vi "DBtest.vi"() -> ()   [LabVIEW 2010]
uses:
  <vilib>/addons/database/Connection.llb/DB Tools Open Connec (Path).vi
  70user.lib/TheSigTab.vi
  <vilib>/addons/database/Connection.llb/Conn Get Properties.vi
  <vilib>/addons/database/NI_Database_API.lvlib
panel:
  out "provider":string
  in  "AllMeasures":cluster{"x0":dbl, "dx":dbl, "y":sgl[][]}[](array[cluster])=[{"x0"=0.0, "dx"=2.011173184357542, "y"=[7.555169582366943, 7.5977783203125, 7.770636558532715, 7.640630722045898, 7.5977783203125, 7.9028544425964355, 7.512796401977539, 7.555169582366943, 7.533955097198486, 7.345677375793457, 7.4496870040893555, 7.640630722045898, 7.491700649261475, 7.387104511260986, 7.576444149017334, 7.263514995574951, 7.512796401977539, 7.576444149017334, 7.263514995574951, 7.814460277557373, 7.662145614624023, 7.512796401977539, 7.3250508308410645, 7.79251766204834, 7.576444149017334, 8.105413436889648, 7.4706645011901855, 7.4496870040893555, 7.407908916473389, 7.705357551574707, 7.6191725730896, 7.555169582366943, 7.345677375793457, 7.662145614624023, 7.662145614624023, 7.4496870040893555, 7.407908916473389, 7.836464881896973, 7.4706645011901855, 7.283968448638916, 7.491700649261475, 7.640630722045898, 7.4496870040893555, 7.662145614624023, 7.705357551574707, 7.533955097198486, 7.283968448638916, 7.9028544425964355, 7.555169582366943, 7.8806633949279785, 7.683721542358398, 7.836464881896973, 7.727055072784424, 7.512796401977539, 7.576444149017334, 7.576444149017334, 7.345677375793457, 7.3250508308410645, 8.105413436889648, 7.79251766204834, 7.345677375793457, 7.304482460021973, 7.407908916473389, 7.081995964050293, 7.491700649261475, 7.141993522644043, 7.640630722045898, 7.243119716644287, 7.141993522644043, 7.5977783203125, 7.512796401977539, 7.345677375793457, 7.4496870040893555, 7.533955097198486, 7.6191725730896, 7.345677375793457, 7.705357551574707, 7.925107955932617, 7.121939182281494, 7.4706645011901855, 7.705357551574707, 7.662145614624023, 7.662145614624023, 7.814460277557373, 7.304482460021973, 7.748816967010498, 7.263514995574951, 7.79251766204834, 7.4496870040893555, 7.705357551574707, 7.5977783203125, 7.407908916473389, 7.576444149017334, 7.512796401977539, 7.533955097198486, 7.5977783203125, 7.683721542358398, 7.8806633949279785, 7.8806633949279785, 7.555169582366943, 7.79251766204834, 7.640630722045898, 7.705357551574707, 7.512796401977539, 7.304482460021973, 7.512796401977539, 7.770636558532715, 8.574320793151855, 7.640630722045898, 7.79251766204834, 7.407908916473389, 7.8806633949279785, 7.533955097198486, 7.814460277557373, 7.576444149017334, 7.99224853515625, 7.79251766204834, 7.491700649261475, 7.814460277557373, 7.662145614624023, 7.640630722045898, 7.748816967010498, 7.683721542358398, 7.662145614624023, 7.79251766204834, 7.79251766204834, 7.6191725730896, 7.79251766204834, 7.770636558532715, 7.79251766204834, 7.748816967010498, 7.4706645011901855, 7.640630722045898, 7.182271957397461, 7.304482460021973, 7.836464881896973, 7.345677375793457, 7.512796401977539, 7.182271957397461, 7.182271957397461, 7.640630722045898, 7.662145614624023, 8.151124954223633, 7.533955097198486, 7.222781181335449, 7.283968448638916, 7.512796401977539, 7.407908916473389, 7.5977783203125, 7.533955097198486, 7.366361618041992, 7.022505283355713, 7.925107955932617, 7.512796401977539, 7.640630722045898, 7.283968448638916, 7.662145614624023, 7.182271957397461, 7.4706645011901855, 7.4496870040893555, 7.4706645011901855, 7.8806633949279785, 7.8806633949279785, 7.533955097198486, 7.533955097198486, 7.5977783203125, 7.4706645011901855, 7.576444149017334, 7.947423934936523, 8.128236770629883, 7.3250508308410645, 7.727055072784424, 7.727055072784424, 7.6191725730896, 7.4706645011901855, 7.533955097198486, 7.555169582366943, 7.683721542358398, 7.576444149017334, 7.770636558532715, 3.1244683265686035, 3.0721945762634277, 3.1865789890289307, 3.2226243019104004, 3.1244683265686035, 3.1332662105560303, 3.195552110671997, 3.168708562850952, 3.2226243019104004, 3.080845594406128, 3.0721945762634277, 3.1420891284942627, 3.0895206928253174, 3.2407989501953125, 3.268254518508911, 3.195552110671997, 3.204550266265869, 3.029301881790161, 3.1332662105560303, 3.314530849456787, 3.399484395980835, 3.159811019897461, 3.1865789890289307, 3.1420891284942627, 3.1332662105560303, 3.380419969558716, 3.3520236015319824, 3.0038535594940186, 3.204550266265869, 3.249924659729004, 3.2959413528442383, 3.195552110671997, 3.195552110671997, 3.168708562850952, 3.159811019897461, 3.0982203483581543, 3.1509368419647217, 3.177631378173828, 3.195552110671997, 3.2135753631591797, 3.231698751449585, 3.1332662105560303, 3.1420891284942627, 3.204550266265869, 3.1509368419647217, 3.2135753631591797, 3.1420891284942627, 3.0635666847229004, 3.204550266265869, 3.1509368419647217, 3.115694761276245, 3.168708562850952, 3.195552110671997, 3.054964303970337, 3.195552110671997, 3.159811019897461, 3.1420891284942627, 3.268254518508911, 3.259077548980713, 3.2959413528442383, 3.0982203483581543, 3.2407989501953125, 3.204550266265869, 3.259077548980713, 3.115694761276245, 3.204550266265869, 3.0982203483581543, 3.323864221572876, 3.204550266265869, 3.1865789890289307, 3.115694761276245, 3.361462354660034, 3.1420891284942627, 3.3520236015319824, 3.2226243019104004, 3.3052237033843994, 3.115694761276245, 3.1865789890289307, 3.177631378173828, 3.159811019897461, 3.0895206928253174, 3.159811019897461, 3.249924659729004, 3.2407989501953125, 3.3520236015319824, 3.249924659729004, 3.1069445610046387, 3.2135753631591797, 3.0895206928253174, 3.4186580181121826, 3.195552110671997, 3.1420891284942627, 3.1332662105560303, 3.2774574756622314, 3.2774574756622314, 3.195552110671997, 3.204550266265869, 3.249924659729004, 3.1244683265686035, 3.1865789890289307, 3.1509368419647217, 3.2407989501953125, 3.2407989501953125, 3.2226243019104004, 3.0635666847229004, 3.195552110671997, 3.361462354660034, 3.3709278106689453, 3.204550266265869, 3.268254518508911, 3.3426096439361572, 3.1865789890289307, 3.333223819732666, 3.231698751449585, 3.249924659729004, 3.204550266265869, 3.1332662105560303, 3.1332662105560303, 3.204550266265869, 3.0982203483581543, 3.0982203483581543, 3.080845594406128, 3.2407989501953125, 3.286686420440674, 3.2135753631591797, 3.333223819732666, 3.204550266265869, 3.0895206928253174, 3.168708562850952, 3.1244683265686035, 3.0635666847229004, 3.168708562850952, 3.3052237033843994, 3.0378317832946777, 3.195552110671997, 3.204550266265869, 3.3052237033843994, 3.1244683265686035, 3.2407989501953125, 3.2407989501953125, 3.0635666847229004, 3.204550266265869, 3.2407989501953125, 3.159811019897461, 3.1865789890289307, 3.159811019897461, 3.0982203483581543, 3.2774574756622314, 3.1865789890289307, 3.1865789890289307, 3.249924659729004, 3.159811019897461, 3.2407989501953125, 3.177631378173828, 3.1420891284942627, 3.159811019897461, 3.168708562850952, 3.168708562850952, 3.2407989501953125, 3.361462354660034, 3.249924659729004, 3.1509368419647217, 3.249924659729004, 3.159811019897461, 3.2774574756622314, 3.1865789890289307, 3.115694761276245, 3.399484395980835, 3.399484395980835, 3.323864221572876, 3.1865789890289307, 3.249924659729004, 3.3520236015319824, 3.231698751449585, 3.080845594406128, 3.177631378173828, 3.231698751449585, 3.195552110671997, 3.168708562850952, 3.2407989501953125, 2.4190430641174316, 2.3919858932495117, 2.4258549213409424, 2.602530002593994, 2.47407865524292, 2.4395363330841064, 2.5303661823272705, 2.4532952308654785, 2.4464058876037598, 2.4464058876037598, 2.365231990814209, 2.432685613632202, 2.4950380325317383, 2.5161752700805664, 2.5879344940185547, 2.6172075271606445, 2.378571033477783, 2.371892213821411, 2.432685613632202, 2.4395363330841064, 2.4464058876037598, 2.4258549213409424, 2.47407865524292, 2.580667018890381, 2.595221757888794, 2.4602034091949463, 2.602530002593994, 2.3519670963287354, 2.4532952308654785, 2.4880316257476807, 2.502063751220703, 2.3919858932495117, 2.365231990814209, 2.4950380325317383, 2.3919858932495117, 2.398721933364868, 2.3585898876190186, 2.41225004196167, 2.4190430641174316, 2.4532952308654785, 2.398721933364868, 2.3852694034576416, 2.502063751220703, 2.4395363330841064, 2.2867507934570312, 2.4671308994293213, 2.371892213821411, 2.5161752700805664, 2.4190430641174316, 2.4464058876037598, 2.3919858932495117, 2.4190430641174316, 2.566194534301758, 2.502063751220703, 2.5879344940185547, 2.378571033477783, 2.573420524597168, 2.3585898876190186, 2.4810452461242676, 2.4054765701293945, 2.365231990814209, 2.3061234951019287, 2.4054765701293945, 2.3453621864318848, 2.3061234951019287, 2.378571033477783, 2.3061234951019287, 2.4464058876037598, 2.312617778778076, 2.432685613632202, 2.378571033477783, 2.41225004196167, 2.365231990814209, 2.4190430641174316, 2.573420524597168, 2.432685613632202, 2.378571033477783, 2.4532952308654785, 2.398721933364868, 2.4810452461242676, 2.432685613632202, 2.5374913215637207, 2.5446372032165527, 2.5161752700805664, 2.4190430641174316, 2.432685613632202, 2.4258549213409424, 2.3519670963287354, 2.4880316257476807, 2.3919858932495117, 2.432685613632202, 2.5091099739074707, 2.41225004196167, 2.378571033477783, 2.4464058876037598, 2.5446372032165527, 2.378571033477783, 2.5232603549957275, 2.580667018890381, 2.3919858932495117, 2.4532952308654785, 2.4671308994293213, 2.5374913215637207, 2.398721933364868, 2.3919858932495117, 2.5091099739074707, 2.4880316257476807, 2.573420524597168, 2.4258549213409424, 2.4880316257476807, 2.432685613632202, 2.398721933364868, 2.4671308994293213, 2.41225004196167, 2.4950380325317383, 2.502063751220703, 2.5374913215637207, 2.551802635192871, 2.432685613632202, 2.3585898876190186, 2.325659990310669, 2.3852694034576416, 2.4190430641174316, 2.398721933364868, 2.4054765701293945, 2.398721933364868, 2.398721933364868, 2.371892213821411, 2.502063751220703, 2.378571033477783, 2.3453621864318848, 2.432685613632202, 2.5879344940185547, 2.2931900024414062, 2.3061234951019287, 2.398721933364868, 2.5161752700805664, 2.332209348678589, 2.3387765884399414, 2.325659990310669, 2.319129705429077, 2.4054765701293945, 2.4395363330841064, 2.4395363330841064, 2.3585898876190186, 2.4671308994293213, 2.47407865524292, 2.312617778778076, 2.3453621864318848, 2.3919858932495117, 2.319129705429077, 2.371892213821411, 2.432685613632202, 2.5232603549957275, 2.4054765701293945, 2.41225004196167, 2.3585898876190186, 2.3453621864318848, 2.325659990310669, 2.41225004196167, 2.4190430641174316, 2.595221757888794, 2.4190430641174316, 2.4532952308654785, 2.3387765884399414, 2.5446372032165527, 2.6393802165985107, 2.47407865524292, 2.4671308994293213, 2.609858512878418, 2.5091099739074707, 2.6468122005462646, 2.5161752700805664, 2.4054765701293945, 2.398721933364868, 2.3919858932495117, 2.4880316257476807, 2.4602034091949463, 2.4880316257476807, 2.3585898876190186]}, ...(5 in all)]
  in  "Table":string[][](table)=[["rty77", "Фаза", "Ch0", "6", "Градусы"], ["rty77", "Фаза", "Ch1", "7", "Градусы"], ["rty77", "Фаза", "Ch2", "1", "Градусы"], ["rty77", "Фаза", "Ch3", "2", "Градусы"], ["rty77", "Фаза", "Ch4", "3", "Градусы"], ["rty77", "Напряжение/Ток", "Ch0", "0,00", "В"], ["rty77", "Напряжение/Ток", "Ch1", "0,00", "В"], ["rty77", "Напряжение/Ток", "Ch2", "0,00", "В"], ["rty77", "Напряжение/Ток", "Ch3", "0,00", "В"], ["rty77", "Напряжение/Ток", "Ch4", "0,00", "В"], ["rty77", "Частота", "Ch0", "300,00", "Гц"]]
  out "Slide":u8(slide) scale=0.0..100.0
  out "error out":errorcluster
  out "tables":string[](array[string])
  in  "connection information":path
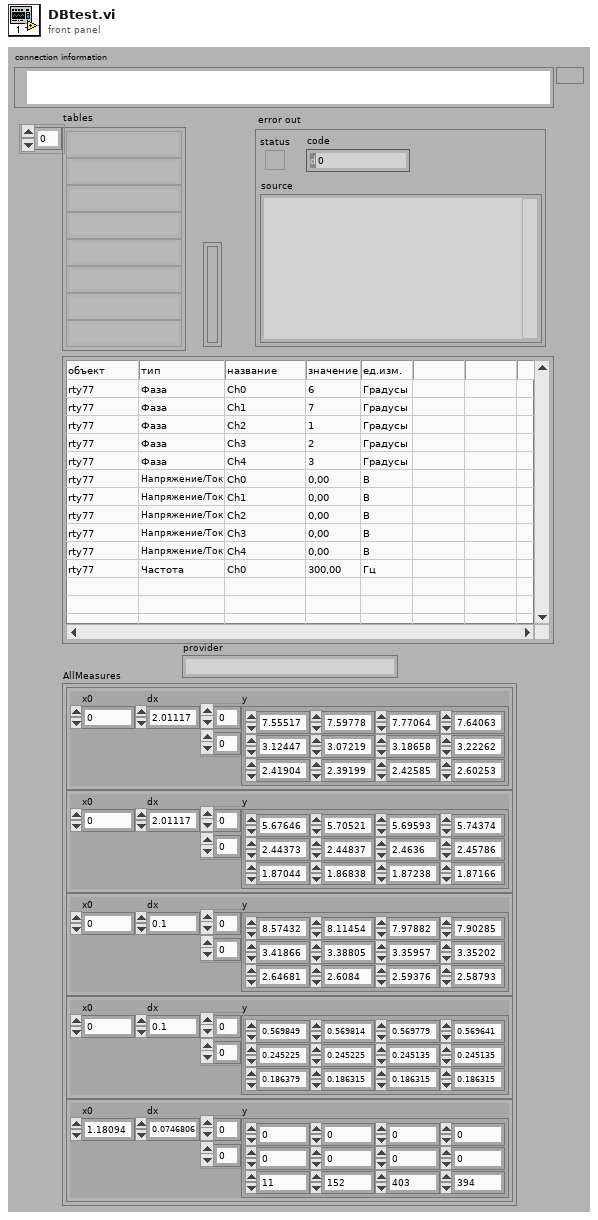
[diagram p1: front panel]
types:
  T1 = typedef "NI_Database_API.lvlib/Conn ObjectReference.ctl" = refnum<k1>
  T2 = cluster{"Сигнал":string, "Тип":enum16{"Напряжение/Ток", "ЧР", "Температура", "Давление"}, "Object":string}[]
  T3 = typedef "NI_Database_API.lvlib/Conn Properties.ctl" = cluster{"command timeout (s)":i32, "connection string":string, "default database":string, "provider":string}
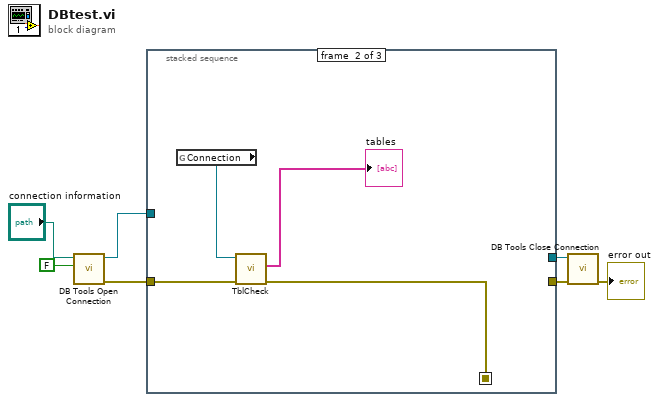
[diagram p0: block diagram]
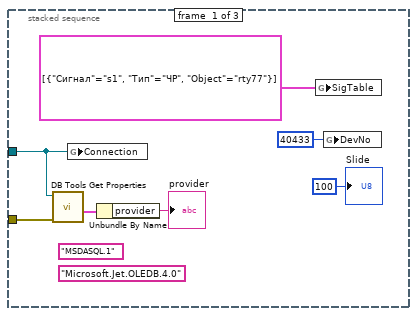
[diagram p2: hidden frame]
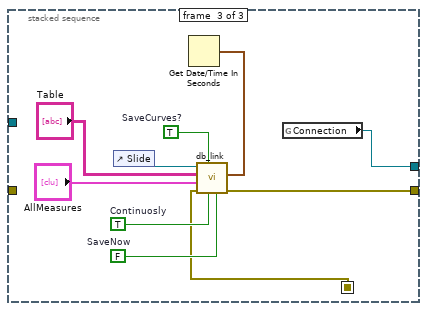
[diagram p3: hidden frame]
diagram:
  n1 = call-poly <vilib>:"DB Tools Open Connection.vi"("prompt? (F)"=FALSE ("prompt? (f)"), "connection information"="connection information") -> ("error out"=w7:errorcluster, "connection reference"=w1:T1)  [unwired: 6 in]
  n2 = stacked-sequence {
    seq-local: [_ w15 _] -> [_ _ w19]
    tunnel: w7 -> [w11 w18 _]
    tunnel: [_ _ w22] -> w5
    tunnel: [_ _ w20] -> w4
    tunnel: w1 -> [w10 _ _]
    frame #0 {
      (unwired) "Microsoft.Jet.OLEDB.4.0"
      (unwired) "MSDASQL.1"
      n3 = call-poly <vilib>:"DB Tools Get Properties.vi"("error in (no error)"=w11, "connection reference"=w10) -> ("connection properties"=w9:T3)  [unwired: 3 in, 2 out]
      n4 = global write "TheSigTab.vi" "Connection"(w10) -> ()
      n5 = Unbundle By Name(w9) -> ("provider"=→"provider":string)
      n6 = global write "TheSigTab.vi" "SigTable"(T2 [{"Сигнал"="s1", "Тип"=enum."ЧР", "Object"="rty77"}] ("SigTable")) -> ()
      n7 = global write "TheSigTab.vi" "DevNo"(u32 40433 ("DevNo")) -> ()
      "Slide" <- u8 100 ("Slide")
    }
    frame #1 {
      n8 = global read "TheSigTab.vi" "Connection"() -> (w16:T1)
      n9 = call "TblCheck.vi"("error in"=w18, "connection reference"=w16) -> ("error out"=w15:errorcluster, "tables"=→"tables":string[])  [unwired: 3 in, 1 out]
    }
    frame #2 {
      w24 = FALSE  # SaveNow
      w25 = TRUE  # Continuosly
      w27 = TRUE  # SaveCurves?
      n10 = control-ref of="Slide"() -> (w26:refnum<vi>)
      n11 = Get Date/Time In Seconds() -> (seconds since 1Jan1904=w28:timestamp)
      n12 = call "db_link.vi"("Current time"=w28, "SaveNow"=w24, "Continuosly"=w25, "SaveCurves?"=w27, "error in"=w19, "AllMeasures"="AllMeasures", "Table"="Table", "reference"=w26) -> ("error"=w20:errorcluster)  [unwired: 3 in]
      n13 = global read "TheSigTab.vi" "Connection"() -> (w22:T1)
    }
  }
  n14 = call <vilib>:"DB Tools Close Connection.vi"("error in (no error)"=w4, "connection reference"=w5) -> ("error out"=→"error out":errorcluster)  [unwired: 5 in]
